vi "Get File Path.vi"(8 "error in (no error)":errorcluster, 11 "queue in":T1) -> (0 "error out":errorcluster, 2 "file path":path, 3 "queue out":T1, 5 "need update":bool)   [LabVIEW 2017, in "NI_LVConfig.lvlib"]
uses:
  <vilib>/Utility/config.llb/NI_LVConfig.lvlib
  <vilib>/Utility/config.llb/Config Queue.ctl
  <vilib>/Utility/config.llb/Config Data.ctl
  <vilib>/Utility/config.llb/Section.ctl
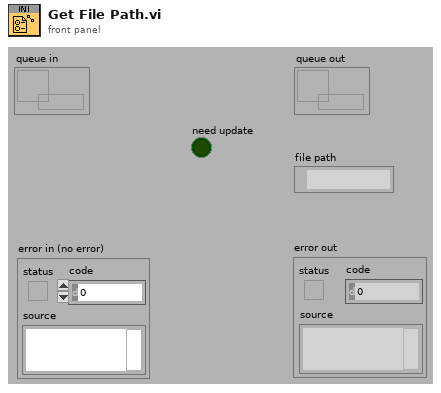
[diagram p1: front panel]
types:
  T1 = typedef "NI_LVConfig.lvlib/Config Queue.ctl" = refnum<queue>
  T2 = typedef "NI_LVConfig.lvlib/Config Data.ctl" = cluster{"sections":T3[], "path":path, "dirty":bool}
  T3 = typedef "NI_LVConfig.lvlib/Section.ctl" = cluster{"name":string, "comment":string, "kvc":string[][]}
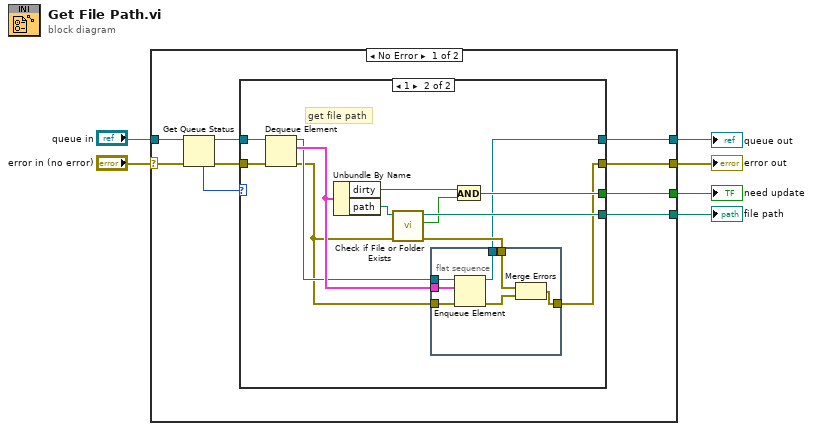
[diagram p0: block diagram]
diagram:
  n1 = case shown="No Error" "error in (no error)" {
    selector: "error in (no error)" -> [w10 w38]
    tunnel: "queue in" -> [w13 w39]
    tunnel: [w15 _] -> w6
    tunnel: [w11 w39] -> w2
    tunnel: [w14 w38] -> w4
    tunnel: [w7 _] -> w1
    frame No Error {
      n2 = Get Queue Status(queue=w13, error in (no error)=w10) -> (queue out=w12:T1, error out=w9:errorcluster, # elements in queue=w8:i32)  [unwired: 1 in, 5 out]
      n3 = case shown="1" w8 {
        tunnel: [_ w27] -> w15
        tunnel: [w16 w19] -> w14
        tunnel: w12 -> [w17 w30]
        tunnel: [w17 w18] -> w11
        tunnel: w9 -> [w16 w29]
        tunnel: [_ w26] -> w7
        frame 0, Default {
        }
        frame 1 {
          # "get file path"
          n4 = Dequeue Element(queue=w30, error in (no error)=w29) -> (queue out=w22:T1, element=w23:T2, error out=w21:errorcluster)  [unwired: 1 in, 1 out]
          n5 = Unbundle By Name(w23) -> ("dirty"=w25:bool, "path"=w28:path)
          n6 = call <vilib>:"Check if File or Folder Exists.vi"("error in (no error)"=w21, "path"=w28) -> ("error out"=w20:errorcluster, "file or folder exists?"=w24:bool, "dup path"=w27:path)  [unwired: 7 out]
          n7 = flat-sequence {
            tunnel: w23 -> [w37]
            tunnel: w22 -> [w36]
            tunnel: w21 -> [w35]
            tunnel: w20 -> [w33]
            tunnel: [w32] -> w19
            tunnel: [w31] -> w18
            frame #0 {
              n8 = Enqueue Element(queue=w36, element=w37, error in (no error)=w35) -> (queue out=w31:T1, error out=w34:errorcluster)  [unwired: 1 in, 1 out]
              n9 = Merge Errors(w33, w34) -> (w32:errorcluster)
            }
          }
          n10 = And(x=w25, y=w24) -> (x .and. y?=w26:bool)
        }
      }
    }
    frame Error {
    }
  }
  "error out" <- w4
  "file path" <- w6
  "queue out" <- w2
  "need update" <- w1
